vi "Stop or Error.vi"(8 "Error In":errorcluster, 9 "Stop Button":bool) -> (0 "Error Out":errorcluster, 1 "Stop or Error?":bool)   [LabVIEW 2013]
doc: "This sub-VI checks whether the main VI stop button has been pressed, or an error has occurred. If either\nhappens, it outputs a boolean True; otherwise False."
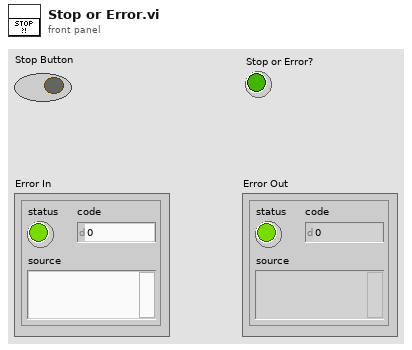
[diagram p1: front panel]
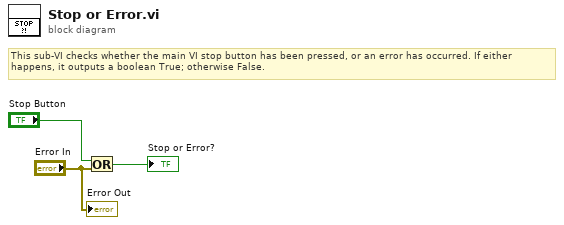
[diagram p0: block diagram]
diagram:
  # "This sub-VI checks whether the main VI stop button has been pressed, or an error has occurred. If either\nhappens, it outputs a boolean True; otherwise False."
  n1 = Or(x="Stop Button", y="Error In") -> (x .or. y?=→"Stop or Error?":bool)
  "Error Out" <- "Error In"
